vi "ArmUpdateLimits.vi"() -> ()   [LabVIEW 2015]
uses:
  LowShooter/Implementation/Shooter Global.vi
  <vilib>/gmath/NI_Gmath.lvlib
panel:
  out "spread value":dbl
  out "subarray":dbl[](array[numeric])
  in  "error in (no error)":errorcluster
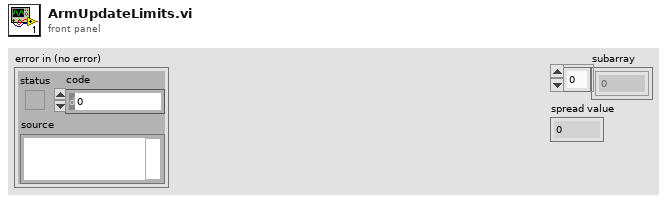
[diagram p1: front panel]
types:
  T1 = typedef "Detailed Motor Type Def.ctl" = cluster{"MotorRef":T2, "Encoder Ticks Per Rev":dbl, "Set Position":dbl, "Wheel Radius":dbl}
  T2 = typedef "WPI_MotorControlDeviceRef.ctl" = cluster{"DeviceStatus":errorcluster, "Type":T3, "PWM":cluster{"PWM Channel":T4, "DeadBand":T5}, "CAN":cluster{"Device Number":u8, "Control Mode":T6, "Semaphore":T7, "Max Vout":dbl, "TalonSRX Control Mode":T8}, "Invert":bool}
  T3 = typedef "WPI_MotorControlType.ctl" = enum16{"PWM", "CAN", "CANTalonSRX"}
  T4 = typedef "FPGA_DIOPWMChannel.ctl" = enum8{"PWM 0", "PWM 1", "PWM 2", "PWM 3", "PWM 4", "PWM 5", "PWM 6", "PWM 7", "PWM 8", "PWM 9", "PWM MXP 0", "PWM MXP 1", "PWM MXP 2", "PWM MXP 3", "PWM MXP 4", "PWM MXP 5", "PWM MXP 6", "PWM MXP 7", "PWM MXP 8", "PWM MXP 9", "Invalid"}
  T5 = typedef "WPI_PWMDeadband.ctl" = cluster{"Name":string, "maxPositivePwm":i32, "minPositivePwm":i32, "centerPwm":i32, "maxNegativePwm":i32, "minNegativePwm":i32, "angularRange":u16}
  T6 = typedef "WPI_CANJaguar_ControlMode.ctl" = enum8{"Percent VBus", "Current", "Speed", "Position", "Voltage"}
  T7 = typedef "Semaphore RefNum" = refnum<k1>
  T8 = typedef "WPI_CANTalonSRX_APIControlMode.ctl" = enum8{"Percent VBus", "Speed", "Position", "Slave", "Unchanged / Invalid", "Voltage Compensation", "Current", "Motion Profile"}
  T9 = typedef "WPI_CANTalonSRX_GlobalStatus.ctl" = cluster{"Applied Throttle":dbl, "Module Enabled":bool, "CAN Error":errorcluster, "Closed Loop Error":dbl, "Forward Limit Switch Closed":bool, "Reverse Limit Switch Closed":bool, "Sensor Position":dbl, "Sensor Velocity":dbl, "Current":dbl, "Sticky Fault - Over Temp":bool, "Sticky Fault - Under Voltage":bool, "Sticky Fault - Forward Limit":bool, "Sticky Fault - Reverse Limit":bool, "Sticky Fault - Forward Soft Limit":bool, "Sticky Fault - Reverse Soft Limit":bool, "Brake is Enabled":bool, "Encoder Position":dbl, "Encoder Velocity":dbl, "Encoder Index Count":dbl, "Encoder A Pin State":bool, "Encoder B Pin State":bool, "Encoder Index Pin State":bool, "Analog In":dbl, "Analog In Velocity":dbl, "Temperature (C)":dbl, "Battery Voltage":dbl, "Control 5 Is Supported":bool, "Current Profile Slot Select":dbl, "Pos Div 8":bool, "Vel Div 4":bool, "Pulse Width Position":i32, "Pulse Width Velocity":i32, "Pulse Width Rise To Rise (us)":i32, "Pulse Width Rise To Fall (us)":i32, "Mot Prof Active Is Under Run":bool, "Mot Prof Active Has Under Run":bool, "Mot Prof Active Is Last":bool, "Mot Prof Active Velocity Only":bool, "Mot Prof Active Is Valid":bool, "Mot Prof Buffer Is Full":bool, "Mot Prof Active Profile Slot Select":i32, "Mot Prof NextID":i32, "Mot Prof Count":i32, "Mot Prof Active Velocity":dbl, "Mot Prof Active Position":dbl, "Mot Prof Output Enable":i32}
  T10 = typedef "Arm Settings Type Def.ctl" = cluster{"Min Arm Pos":dbl, "Max Arm Pos":dbl, "Drive Pos":dbl, "Arm Increments":dbl, "Obstacle Pos":dbl, "Max Current":dbl}
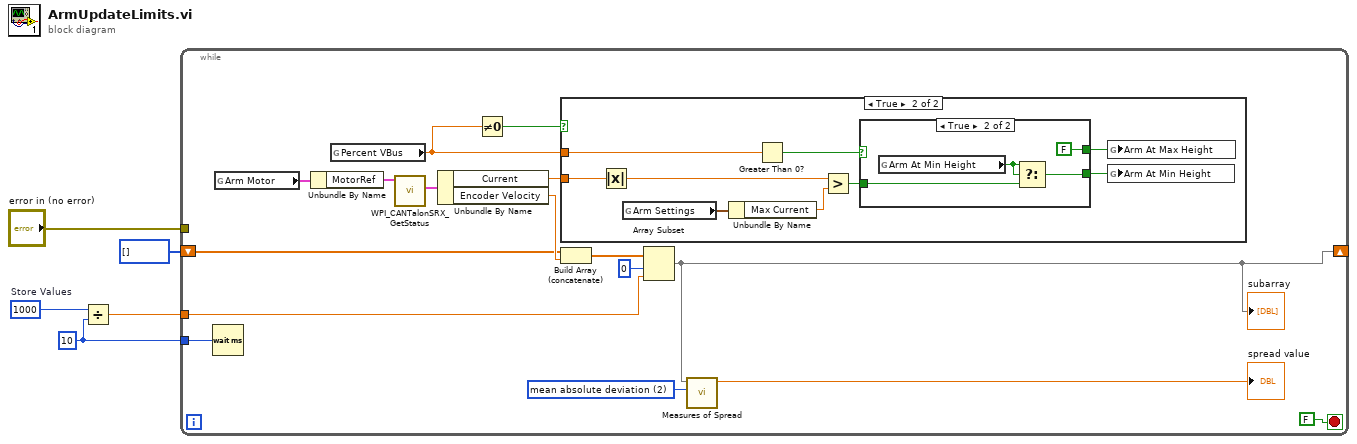
[diagram p0: block diagram]
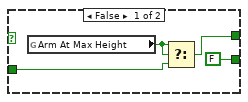
[diagram p3: hidden frame]
diagram:
  w2 = u32 10 ("milliseconds to wait")
  w3 = 1000  # Store Values
  n1 = Divide(x=w3, y=w2) -> (x/y=w1:dbl)
  n2 = while {
    tunnel: "error in (no error)" -> [_]
    shift-right: [w7] -> _
    shift-left: i32[] [] -> [w13]
    tunnel: w2 -> [w12]
    tunnel: w1 -> [w9]
    stop <- FALSE stop-if-true
    w8 = 2 items=["standard deviation", "range", "mean absolute deviation", "interquartile range"] ("type")
    n3 = Wait (ms)(milliseconds to wait=w12) -> ()  [unwired: 1 out]
    n4 = global read "Shooter Global.vi" "Arm Motor"() -> (w17:T1)
    n5 = Unbundle By Name(w17) -> ("MotorRef"=w18:T2)
    n6 = global read "Shooter Global.vi" "Percent VBus"() -> (w19:dbl)
    n7 = call <vilib>:"WPI_CANTalonSRX_GetStatus.vi"("CAN Talon SRX Ref"=w18) -> ("Talon SRX Status"=w16:T9)  [unwired: 8 in, 2 out]
    n8 = Unbundle By Name(w16) -> ("Current"=w15:dbl, "Encoder Velocity"=w14:dbl)
    n9 = Not Equal To 0?(x=w19) -> (x != 0?=w21:bool)
    n10 = case shown="True" w21 {
      tunnel: w19 -> [_ w30]
      tunnel: w15 -> [_ w22]
      frame False {
      }
      frame True {
        n11 = Absolute Value(x=w22) -> (abs(x)=w27:dbl)
        n12 = global read "Shooter Global.vi" "Arm Settings"() -> (w28:T10)
        n13 = Unbundle By Name(w28) -> ("Max Current"=w26:dbl)
        n14 = Greater Than 0?(x=w30) -> (x > 0?=w29:bool)
        n15 = Greater?(x=w27, y=w26) -> (0:w24:bool)
        n16 = case shown="True" w29 {
          tunnel: [FALSE ("Arm At Min Height") w37] -> w25
          tunnel: w24 -> [w32 w36]
          tunnel: [w33 FALSE] -> w23
          frame False {
            n17 = global read "Shooter Global.vi" "Arm At Max Height"() -> (w34:bool)
            n18 = Select(t=w34, s=w34, f=w32) -> (s? t:f=w33:bool)
          }
          frame True {
            n19 = global read "Shooter Global.vi" "Arm At Min Height"() -> (w38:bool)
            n20 = Select(t=w38, s=w38, f=w36) -> (s? t:f=w37:bool)
          }
        }
        n21 = global write "Shooter Global.vi" "Arm At Max Height"(w23) -> ()
        n22 = global write "Shooter Global.vi" "Arm At Min Height"(w25) -> ()
      }
    }
    n23 = Build Array (concatenate)(w13, w14) -> (w11:dbl[])
    n24 = Array Subset(array=w11, index=0, length=w9) -> (w7:dbl[])
    "subarray" <- w7
    n25 = call <vilib>:"Measures of Spread.vi"("type"=w8, "x array"=w7) -> ("spread value"=→"spread value":dbl)  [unwired: 8 in, 1 out]
  }
